vi "New Targets Update from Targets Message.vi"(2 "error in":errorcluster, 3 "Targets Message":T2={"type"="", "message"={"capturedAgoMs"=0, "targets"=[{"x"=0.0, "y"=0.0, "z"=0.0, "theta"=0.0}]}}, 4 "Current Time (ms)":dbl) -> (0 "error out":errorcluster, 1 "Targets Update":T1)   [LabVIEW 2016]
uses:
  Targets Message.ctl
  Targets Info.ctl
  Targets Update.ctl
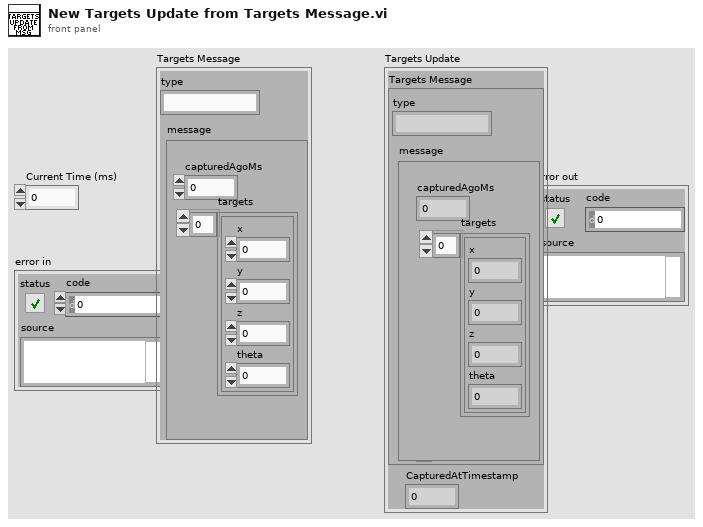
[diagram p1: front panel]
types:
  T1 = typedef "Targets Update.ctl" = cluster{"Valid?":bool, "CapturedAtTimestamp":dbl, "Targets Message":T2}
  T2 = typedef "Targets Message.ctl" = cluster{"type":string, "message":cluster{"capturedAgoMs":i32, "targets":T3[]}}
  T3 = typedef "Targets Info.ctl" = cluster{"x":dbl, "y":dbl, "z":dbl, "theta":dbl}
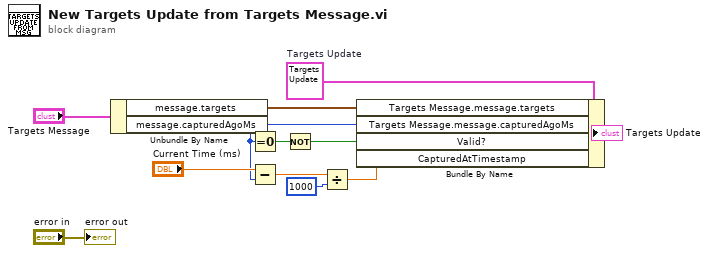
[diagram p0: block diagram]
diagram:
  w3 = T1 {"Valid?"=FALSE, "CapturedAtTimestamp"=0.0, "Targets Message"={"type"="", "message"={"capturedAgoMs"=0, "targets"=[{"x"=0.0, "y"=0.0, "z"=0.0, "theta"=0.0}]}}}  # Targets Update
  n1 = Unbundle By Name("Targets Message") -> ("message.targets"=w2:T3[], "message.capturedAgoMs"=w6:i32)
  n2 = Equal To 0?(x=w6) -> (x = 0?=w12:bool)
  n3 = Subtract(x="Current Time (ms)", y=w6) -> (x-y=w10:dbl)
  n4 = Not(x=w12) -> (.not. x?=w7:bool)
  n5 = Divide(x=w10, y=1000) -> (x/y=w5:dbl)
  n6 = Bundle By Name(cluster=w3, "Targets Message.message.targets"=w2, "Targets Message.message.capturedAgoMs"=w6, "Valid?"=w7, "CapturedAtTimestamp"=w5) -> (→"Targets Update":T1)
  "error out" <- "error in"
